vi "Write bit.vi"(8 "error in":errorcluster, 10 "bit":i32, 11 "Profibus channel in":refnum<class "Profibus channel.lvclass">) -> (0 "error out":errorcluster, 3 "Profibus channel out":refnum<class "Profibus channel.lvclass">)   [LabVIEW 2013, in "Profibus channel.lvclass"]
uses:
  Profibus channel.lvclass
  Profibus channel.lvclass/Profibus channel.ctl
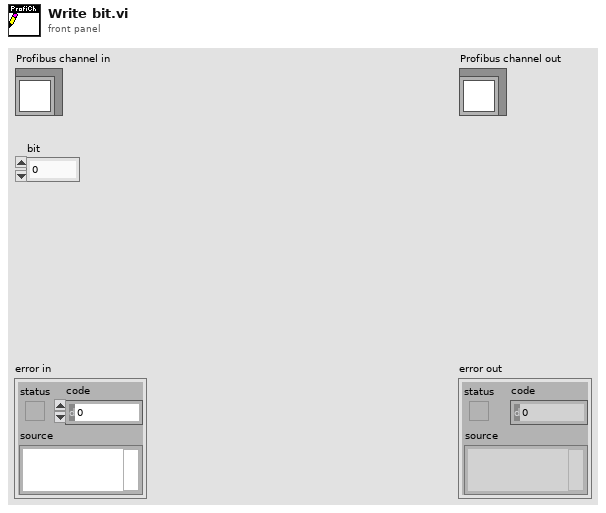
[diagram p1: front panel]
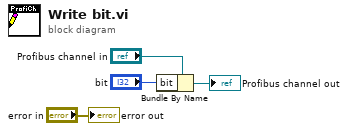
[diagram p0: block diagram]
diagram:
  n1 = Bundle By Name(cluster="Profibus channel in", "bit"="bit") -> (→"Profibus channel out":refnum<class "Profibus channel.lvclass">)
  "error out" <- "error in"
